vi "Launch Project Scanner.vi"(8 "error in (no error)":errorcluster, 11 "Project Ref":refnum<vi>) -> (0 "error out":errorcluster, 3 "Project Ref Out":refnum<vi>)   [LabVIEW 2014]
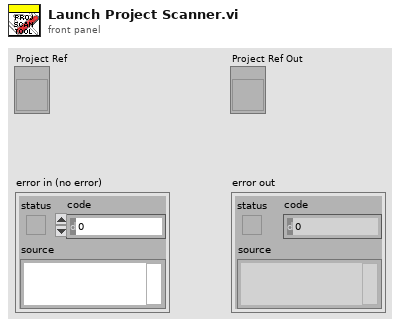
[diagram p1: front panel]
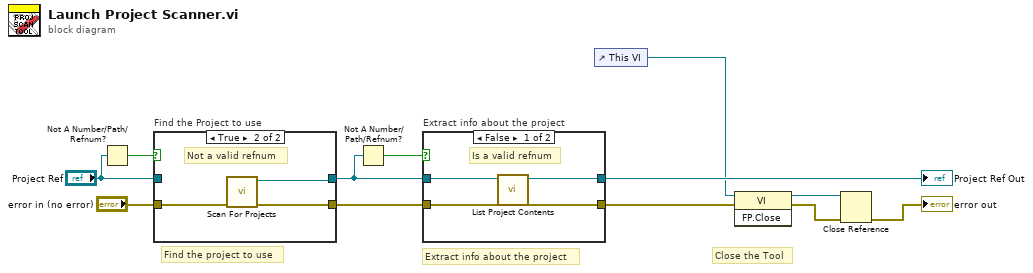
[diagram p0: block diagram]
diagram:
  # "Close the Tool"
  # "Extract info about the project"
  # "Find the project to use"
  n1 = Not A Number/Path/Refnum?(number/path/refnum="Project Ref") -> (NaN/Path/Refnum?=w12:bool)
  n2 = case "Find the Project to use" shown="True" w12 {
    tunnel: "Project Ref" -> [w14 _]
    tunnel: [w14 w17] -> w8
    tunnel: "error in (no error)" -> [w13 w16]
    tunnel: [w13 w15] -> w9
    frame False {
      # "Is a valid refnum"
    }
    frame True {
      # "Not a valid refnum"
      n3 = call "Scan For Projects.vi"("error in (no error)"=w16) -> ("error out"=w15:errorcluster, "Selected Project"=w17:refnum<vi>)  [unwired: 9 in]
    }
  }
  n4 = Not A Number/Path/Refnum?(number/path/refnum=w8) -> (NaN/Path/Refnum?=w7:bool)
  n5 = case "Extract info about the project" shown="False" w7 {
    tunnel: w8 -> [w18 w21]
    tunnel: [w19 w21] -> w5
    tunnel: w9 -> [w20 w22]
    tunnel: [w20 w22] -> w6
    frame False {
      # "Is a valid refnum"
      n6 = call "List Project Contents.vi"("Selected Project"=w18) -> ("Selected Project Out"=w19:refnum<vi>)  [unwired: 10 in]
    }
    frame True {
      # "Not a valid refnum"
    }
  }
  "Project Ref Out" <- w5
  n7 = control-ref of="This VI"() -> (w3:refnum<vi>)
  n8 = invoke class="VI" method="FP.Close"(reference=w3, error in=w6) -> (reference out=w1:refnum<vi>, error out=w4:errorcluster)  [unwired: 1 in, 1 out]
  n9 = Close Reference(reference=w1, error in (no error)=w4) -> (error out=→"error out":errorcluster)
